vi "ConfigureDigitalInputs.vi"(0 "axis in":cluster{"keyHandle":u32, "nodeId":u16}={"keyHandle"=0, "nodeId"=1}, 5 "digital input configuration":T1={"digitalInputNumber"=1, "configuration"=15, "mask"=1, "polarity"=0, "executionMask"=1} {"executionMask" items=["Disabled", "Enabled"]; "polarity" items=["HighActive", "LowActive"]; "mask" items=["Disabled", "Enabled"]; "configuration" items=["Negative Limit Switch"=0, "Positive Limit Switch"=1, "Home Switch"=2, "Position Marker"=3, "Enable"=4, "General Purpose A"=15, "General Purpose B"=14, "General Purpose C"=13, "General Purpose D"=12, "General Purpose E"=11, "General Purpose F"=10, "General Purpose G"=9, "General Purpose H"=8]}, 11 "error in (no error)":errorcluster) -> (4 "axis out":cluster{"keyHandle":u32, "nodeId":u16}={"keyHandle"=0, "nodeId"=1}, 15 "error out":errorcluster)   [LabVIEW 2017, in "maxonEPOS.lvlib"]
doc: "<B>ConfigureDigitalInputs</B> writes the configuration parameters for a digital input to the device."
uses:
  Examples/maxonEPOS.lvlib
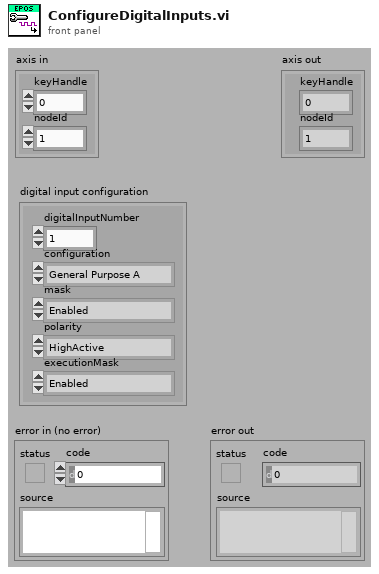
[diagram p1: front panel]
types:
  T1 = cluster{"digitalInputNumber":u16, "configuration":u16, "mask":i32, "polarity":i32, "executionMask":i32}
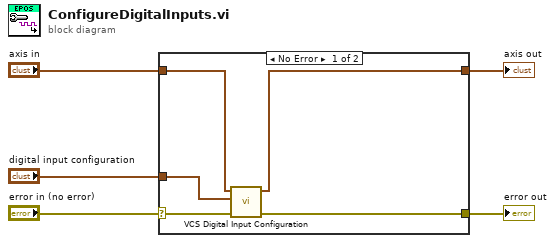
[diagram p0: block diagram]
diagram:
  n1 = case shown="No Error" "error in (no error)" {
    selector: "error in (no error)" -> [w10 w12]
    tunnel: [w6 w12] -> w4
    tunnel: [w7 w11] -> w3
    tunnel: "axis in" -> [w9 w11]
    tunnel: "digital input configuration" -> [w8 _]
    frame No Error {
      n2 = call "VCS Digital Input Configuration.vi"("error in (no error)"=w10, "input configuration"=w8, "axis in"=w9) -> ("error out"=w6:errorcluster, "axis out"=w7:cluster{"keyHandle":u32, "nodeId":u16})  [unwired: 7 in]
    }
    frame Error {
    }
  }
  "error out" <- w4
  "axis out" <- w3
